vi "Build One Term Numeric Functions - Float Types.vi"(11 "Comparison Name":string) -> ()   [LabVIEW 2021]
uses:
  <vilib>/numeric/LVNumericRepresentation.ctl
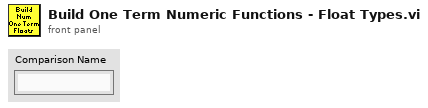
[diagram p1: front panel]
types:
  T1 = typedef "LVNumericRepresentation.ctl" = enum32{"Extended Precision", "Double Precision", "Single Precision", "Long", "Word", "Byte", "Unsigned Long", "Unsigned Word", "Unsigned Byte", "Complex Extended", "Complex Double", "Complex Single", "Quad", "Unsigned Quad", "Fixed-Point"}
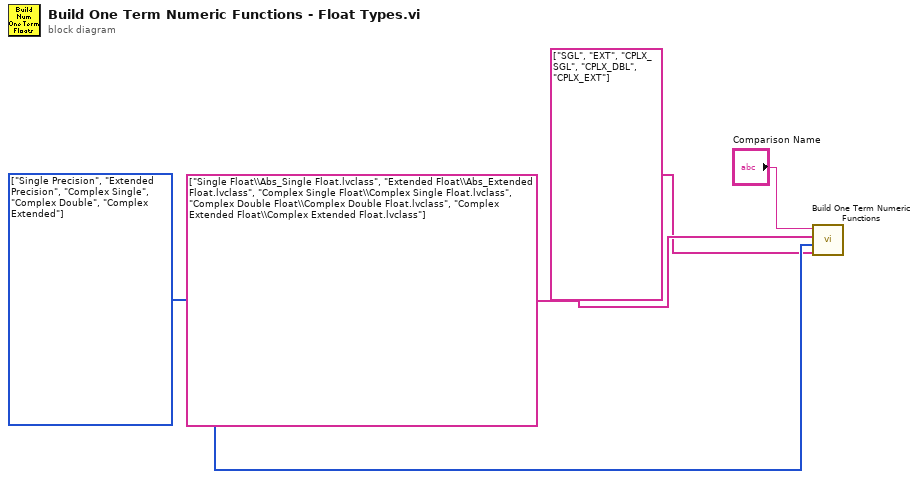
[diagram p0: block diagram]
diagram:
  w3 = T1[] [enum."Single Precision", enum."Extended Precision", enum."Complex Single", enum."Complex Double", enum."Complex Extended"] items=["Extended Precision", "Double Precision", "Single Precision", "Long", "Word", "Byte", "Unsigned Long", "Unsigned Word", "Unsigned Byte", "Complex Extended", "Complex Double", "Complex Single", "Quad", "Unsigned Quad", "Fixed-Point"] ("Representation")
  n1 = call "Build One Term Numeric Functions.vi"("Names"=string[] ["SGL", "EXT", "CPLX_SGL", "CPLX_DBL", "CPLX_EXT"], "Representation"=w3, "Abstract Type Locations"=string[] ["Single Float\\Abs_Single Float.lvclass", "Extended Float\\Abs_Extended Float.lvclass", "Complex Single Float\\Complex Single Float.lvclass", "Complex Double Float\\Complex Double Float.lvclass", "Complex Extended Float\\Complex Extended Float.lvclass"], "Comparison Name"="Comparison Name") -> ()  [unwired: 8 in]
